vi "_Write.vi"(8 "error in (no error)":errorcluster, 10 "Data":string, 11 "WebsocketStream in":refnum<class "WebsocketStream.lvclass">) -> (0 "error out":errorcluster, 3 "WebsocketStream out":refnum<class "WebsocketStream.lvclass">)   [LabVIEW 2020, in "Stream-Websocket.lvlib" / "WebsocketStream.lvclass"]
uses:
  WebsocketStream.lvclass
  OpCode.ctl
  Stream-Websocket.lvlib
  Lock Type.ctl
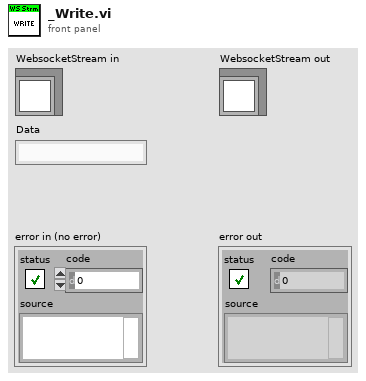
[diagram p1: front panel]
types:
  T1 = typedef "Stream-Websocket.lvlib/WebsocketStream.lvclass/Lock Type.ctl" = enum16{"Read", "Write"}
  T2 = typedef "Stream-Websocket.lvlib/OpCode.ctl" = enum8{"Continuation", "Text", "Binary", "Reserved3", "Reserved4", "Reserved5", "Reserved6", "Reserved7", "Close", "Ping", "Pong", "ReservedB", "ReservedC", "ReservedD", "ReservedE", "ReservedF"}
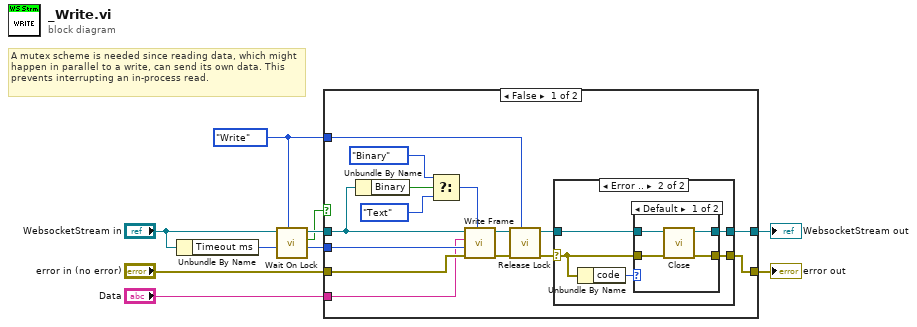
[diagram p0: block diagram]
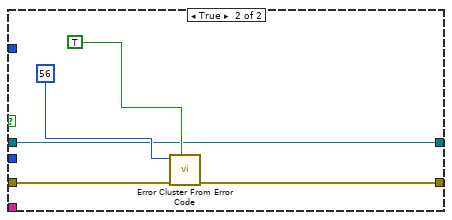
[diagram p4: hidden frame]
diagram:
  w1 = Lock_Type."Write" ("Lock Type")
  # "A mutex scheme is needed since reading data, which might happen in parallel to a write, can send its own data. This prevents interrupting an in-process read."
  n1 = Unbundle By Name("WebsocketStream in") -> ("Timeout ms"=w8:i32)
  n2 = call "Wait On Lock.vi"("Lock Type"=w1, "Timeout ms"=w8, "WebsocketStream in"="WebsocketStream in") -> ("Remaining  Timeout"=w9:i32, "Timeout"=w7:bool, "WebsocketStream out"=w10:refnum<class "WebsocketStream.lvclass">)  [unwired: 5 in, 1 out]
  n3 = case shown="False" w7 {
    tunnel: [w17 w39] -> w4
    tunnel: [w16 w40] -> w3
    tunnel: w10 -> [w15 w39]
    tunnel: w9 -> [w25 _]
    tunnel: "error in (no error)" -> [w24 w43]
    tunnel: "Data" -> [w23 _]
    tunnel: w1 -> [w20 _]
    frame False {
      n4 = Unbundle By Name(w15) -> ("Binary"=w14:bool)
      n5 = Select(t=OpCode."Binary" ("OpCode"), s=w14, f=OpCode."Text" ("OpCode")) -> (s? t:f=w11:T2)
      n6 = call "Write Frame.vi"("OpCode"=w11, "error in (no error)"=w24, "Timeout ms"=w25, "Payload"=w23, "WebsocketStream in"=w15) -> ("error out"=w22:errorcluster, "WebsocketStream out"=w21:refnum<class "WebsocketStream.lvclass">)  [unwired: 4 in, 1 out]
      n7 = call "Release Lock.vi"("Lock Type"=w20, "error in (no error)"=w22, "WebsocketStream in"=w21) -> ("error out"=w19:errorcluster, "WebsocketStream out"=w18:refnum<class "WebsocketStream.lvclass">)  [unwired: 7 in]
      n8 = case shown="Error .." w19 {
        selector: w19 -> [w26 w31]
        tunnel: w18 -> [w27 w28]
        tunnel: [w27 w29] -> w17
        tunnel: [w26 w30] -> w16
        frame No Error {
        }
        frame Error {
          n9 = Unbundle By Name(w31) -> ("code"=w32:i32)
          n10 = case shown="Default" w32 {
            tunnel: w31 -> [w35 w38]
            tunnel: [w34 w38] -> w30
            tunnel: [w33 w37] -> w29
            tunnel: w28 -> [w36 w37]
            frame Default {
              n11 = call-dynamic "Close.vi"("error in (no error)"=w35, "WebsocketStream in"=w36) -> ("error out"=w34:errorcluster, "WebsocketStream out"=w33:refnum<class "WebsocketStream.lvclass">)  [unwired: 8 in]
            }
            frame 56 {
            }
          }
        }
      }
    }
    frame True {
      n12 = call <vilib>:"Error Cluster From Error Code.vi"("show call chain? (False)"=TRUE, "error in (no error)"=w43, "error code (0)"=56) -> ("error out"=w40:errorcluster)  [unwired: 6 in]
    }
  }
  "error out" <- w3
  "WebsocketStream out" <- w4
